vi "Linear Programming Simplex Method.vi"(0 "C":dbl[](array[numeric]) format="%.2f", 1 "M":dbl[][](array[numeric]) format="%.2f", 2 "B":dbl[](array[numeric]) format="%.2f") -> (3 "maximum":dbl format="%.2f", 4 "X":dbl[](array[numeric]) format="%.2f", 5 "ticks":u32, 6 "error":i32)   [LabVIEW 2020, in "NI_Gmath.lvlib"]
doc: "Determines the solution of a linear programming problem."
uses:
  <vilib>/gmath/NI_Gmath.lvlib
panel:
  # "c.x=max!\nm.x>=b\nx>=0"
  # "Example:\n\n C: (1,1) \n M: ((-1,-2))\n B: (-1)"
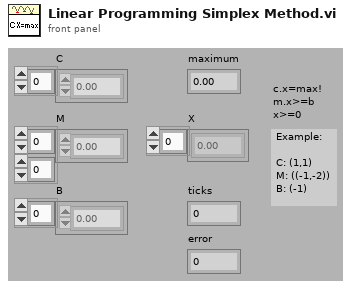
[diagram p1: front panel]
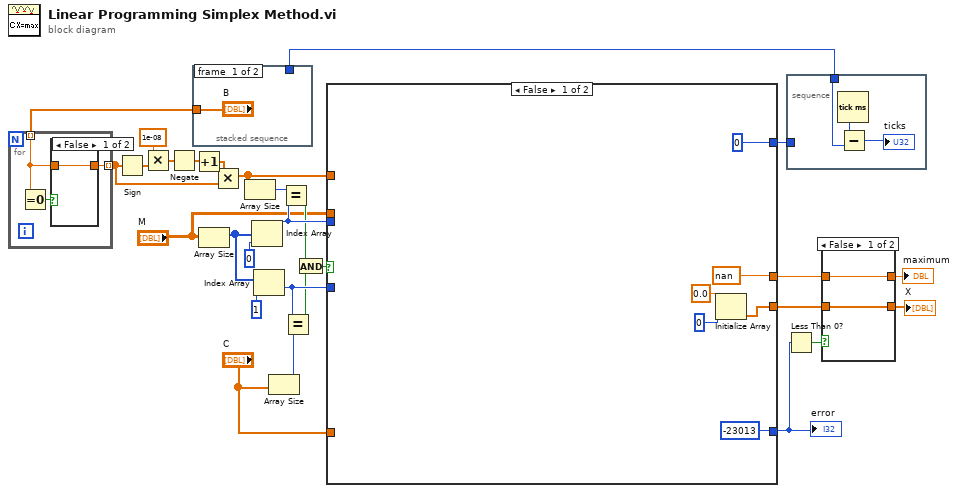
[diagram p0: block diagram]
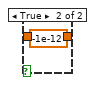
[diagram p2: hidden frame]
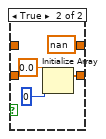
[diagram p3: hidden frame]
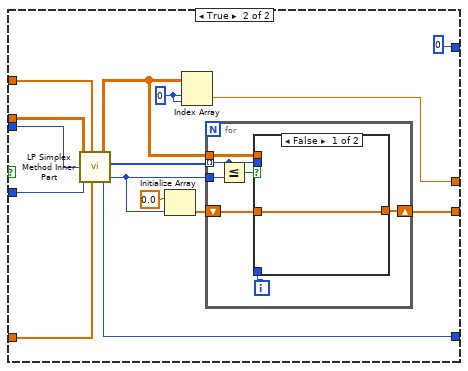
[diagram p4: hidden frame]
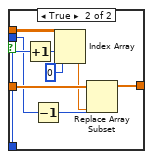
[diagram p5: hidden frame]
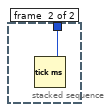
[diagram p6: hidden frame]
diagram:
  n1 = stacked-sequence {
    tunnel: [_ w30] -> w25
    tunnel: ["B" _] -> w1
    frame #0 {
    }
    frame #1 {
      n2 = Tick Count (ms)() -> (millisecond timer value=w30:u32)
    }
  }
  n3 = for {
    tunnel: [w32] -> w3 mode=indexing
    tunnel: w1 -> [w31] mode=indexing
    n4 = Equal To 0?(x=w31) -> (x = 0?=w33:bool)
    n5 = case shown="False" w33 {
      tunnel: w31 -> [w34 _]
      tunnel: [w34 -1e-12] -> w32
      frame False {
      }
      frame True {
      }
    }
  }
  n6 = Sign(1:w3) -> (0:w8:dbl[])
  n7 = Multiply(x=1e-08, y=w8) -> (x*y=w7:dbl[])
  n8 = Negate(x=w7) -> (-x=w6:dbl[])
  n9 = Increment(x=w6) -> (x+1=w5:dbl[])
  n10 = Array Size(array="M") -> (size(s)=w27:i32[])
  n11 = Multiply(x=w5, y=w3) -> (x*y=w4:dbl[])
  n12 = Array Size(array=w4) -> (size(s)=w22:i32)
  n13 = Index Array(array=w27, index=0) -> (element=w21:i32)
  n14 = Index Array(array=w27, index=1) -> (element=w19:i32)
  n15 = Array Size(array="C") -> (size(s)=w20:i32)
  n16 = Equal?(x=w22, y=w21) -> (x = y?=w18:bool)
  n17 = Equal?(x=w19, y=w20) -> (x = y?=w17:bool)
  n18 = And(x=w18, y=w17) -> (x .and. y?=w16:bool)
  n19 = case shown="False" w16 {
    tunnel: "C" -> [_ w52]
    tunnel: w19 -> [_ w49]
    tunnel: w21 -> [_ w48]
    tunnel: w4 -> [_ w47]
    tunnel: "M" -> [_ w46]
    tunnel: [nan w45] -> w13
    tunnel: [w38 w44] -> w11
    tunnel: [0 0] -> w24
    tunnel: [-23013 w43] -> w15
    frame False {
      n20 = Initialize Array(0.0, 0) -> (w38:dbl[])
    }
    frame True {
      w50 = 0
      n21 = call <vilib>:"LP Simplex Method Inner Part.vi"("M"=w46, "B modified"=w47, "first length M"=w48, "second length M"=w49, "C"=w52) -> ("table*"=w56:dbl[][], "m*"=w54:u32[], "length of array"=w55:i32, "error"=w43:i32)
      n22 = Initialize Array(0.0, w55) -> (w53:dbl[])
      n23 = Index Array(array=w56, index (row)=w50, index (col)=w50) -> (element=w45:dbl)
      n24 = for {
        shift-right: [w60] -> w44
        shift-left: w53 -> [w61]
        tunnel: w54 -> [w58] mode=indexing
        tunnel: w55 -> [w63]
        tunnel: w56 -> [w59]
        i -> [w57]
        n25 = Less Or Equal?(x=w58, y=w63) -> (x <= y?=w62:bool)
        n26 = case shown="False" w62 {
          tunnel: w61 -> [w64 w73]
          tunnel: [w64 w72] -> w60
          tunnel: w59 -> [_ w71]
          tunnel: w58 -> [_ w67]
          tunnel: w57 -> [_ w68]
          frame False {
          }
          frame True {
            n27 = Increment(x=w68) -> (x+1=w66:i32)
            n28 = Decrement(x=w67) -> (x-1=w65:u32)
            n29 = Index Array(array=w71, index (row)=w66, index (col)=0) -> (element=w69:dbl)
            n30 = Replace Array Subset(array=w73, new element=w69, index=w65) -> (w72:dbl[])
          }
        }
      }
    }
  }
  "error" <- w15
  n31 = Less Than 0?(x=w15) -> (x < 0?=w14:bool)
  n32 = stacked-sequence {
    tunnel: w25 -> [w74]
    tunnel: w24 -> [_]
    frame #0 {
      n33 = Tick Count (ms)() -> (millisecond timer value=w76:u32)
      n34 = Subtract(x=w76, y=w74) -> (x-y=→"ticks":u32)
    }
  }
  n35 = case shown="False" w14 {
    tunnel: w13 -> [w78 _]
    tunnel: [w78 nan] -> w12
    tunnel: w11 -> [w77 _]
    tunnel: [w77 w79] -> w10
    frame False {
    }
    frame True {
      n36 = Initialize Array(0.0, 0) -> (w79:dbl[])
    }
  }
  "maximum" <- w12
  "X" <- w10
